vi "Sort Robots.vi"(11 "robots_blue":T1[](array[typedef]) {"height" format="%+4.3f"; "pixel_y" format="%+4.3f"; "pixel_x" format="%+4.3f"; "orientation" format="%+4.3f"; "y" format="%+4.3f"; "confidence" format="%4.3f"; "x" format="%+4.3f"}) -> (3 "Array":T1[](array[typedef]) {"height" format="%+4.3f"; "pixel_y" format="%+4.3f"; "pixel_x" format="%+4.3f"; "orientation" format="%+4.3f"; "y" format="%+4.3f"; "confidence" format="%4.3f"; "x" format="%+4.3f"})   [LabVIEW 2017]
uses:
  SSL Detection Robot.ctl
  <vilib>/Analysis/Matrix/Datatypes/RealMatrix.ctl
  <vilib>/Analysis/Matrix/NI_Matrix.lvlib
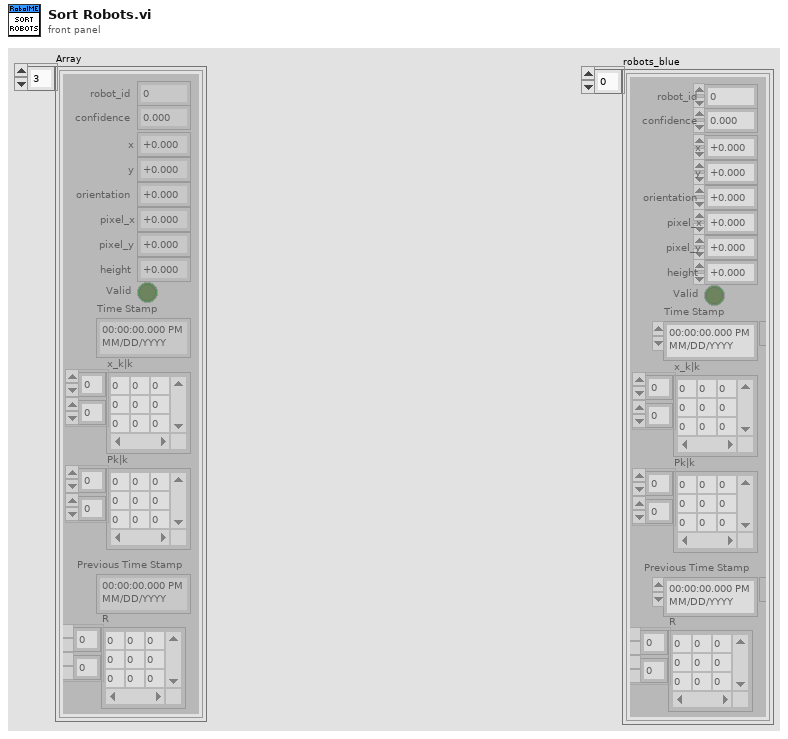
[diagram p1: front panel]
types:
  T1 = typedef "SSL Detection Robot.ctl" = cluster{"x":sgl, "robot_id":u32, "confidence":sgl, "y":sgl, "orientation":sgl, "pixel_x":sgl, "pixel_y":sgl, "height":sgl, "Valid":bool, "Time Stamp":timestamp, "x_k|k":T2, "Pk|k":T2, "Previous Time Stamp":timestamp, "R":T2}
  T2 = typedef "NI_Matrix.lvlib/RealMatrix.ctl" = dbl[][]
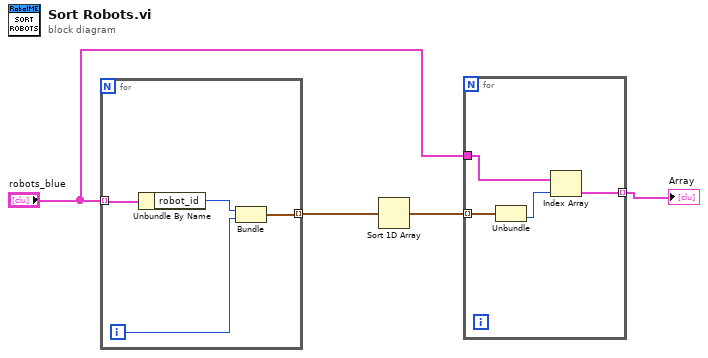
[diagram p0: block diagram]
diagram:
  n1 = for {
    tunnel: "robots_blue" -> [w8] mode=indexing
    tunnel: [w5] -> w4 mode=indexing
    i -> [w6]
    n2 = Unbundle By Name(w8) -> ("robot_id"=w7:u32)
    n3 = Bundle("robot_id"=w7, w6) -> (w5:cluster{"robot_id":u32, i32})  [unwired: 1 in]
  }
  n4 = Sort 1D Array(array=w4) -> (sorted array=w3:cluster{"robot_id":u32, i32}[])
  n5 = for {
    tunnel: w3 -> [w11] mode=indexing
    tunnel: "robots_blue" -> [w12]
    tunnel: [w9] -> w2 mode=indexing
    n6 = Unbundle(w11) -> (w10:i32)  [unwired: 1 out]
    n7 = Index Array(array=w12, index=w10) -> (element=w9:T1)
  }
  "Array" <- w2
